vi "IND560 Serial Read.vi"(8 "error in (no error)":errorcluster, 11 "VISA Refnum in":refnum<visa-resource-name>) -> (0 "error out":errorcluster, 1 "Net Weight":dbl, 2 "IND560 Serial Data":string[][](array[string]), 3 "VISA Refnum out":refnum<visa-resource-name>)   [LabVIEW 2018]
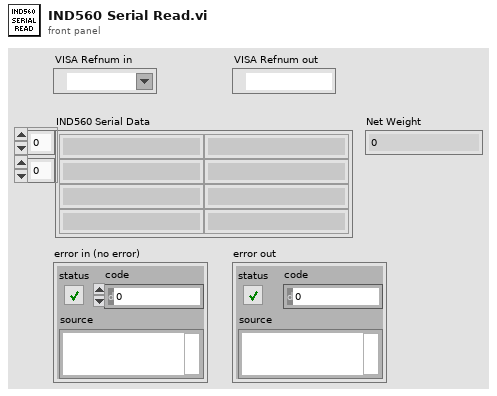
[diagram p1: front panel]
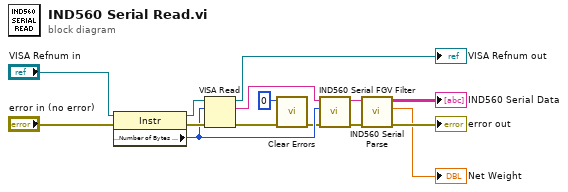
[diagram p0: block diagram]
diagram:
  n1 = property class="Instr"(reference="VISA Refnum in", error in="error in (no error)") -> (reference out=w13:refnum<visa-resource-name>, error out=w12:errorcluster, "Serial Settings:Number of Bytes at Serial Port"=w8:u32)
  n2 = VISA Read(VISA resource name=w13, byte count=w8, error in (no error)=w12) -> (VISA resource name out=→"VISA Refnum out":refnum<visa-resource-name>, read buffer=w7:string, error out=w10:errorcluster)  [unwired: 1 out]
  n3 = call <vilib>:"Clear Errors.vi"("error in (no error)"=w10, "specific error code to clear (0: all)"=0) -> ("error out"=w3:errorcluster)  [unwired: 4 in, 1 out]
  n4 = call "IND560 Serial FGV Filter.vi"("Error In"=w3, "Bytes at Port"=w8, "Weight Template"=w7) -> ("Error Out"=w4:errorcluster, "Filtered Weight"=w6:string)  [unwired: 7 in]
  n5 = call "IND560 Serial Parse.vi"("Error In"=w4, "Weight Template"=w6) -> ("Error Out"=→"error out":errorcluster, "Net Weight"=→"Net Weight":dbl, "IND560 Serial Data"=→"IND560 Serial Data":string[][])  [unwired: 7 in]
